vi "RMS.vi"(11 "current waveform":waveform(dbl)) -> (3 "RMS":dbl)   [LabVIEW 2017]
uses:
  <vilib>/measure/madcrms.llb/Basic Averaged DC-RMS for 1 Chan.vi
  <vilib>/measure/NI_MAPro.lvlib
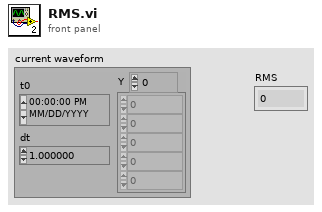
[diagram p1: front panel]
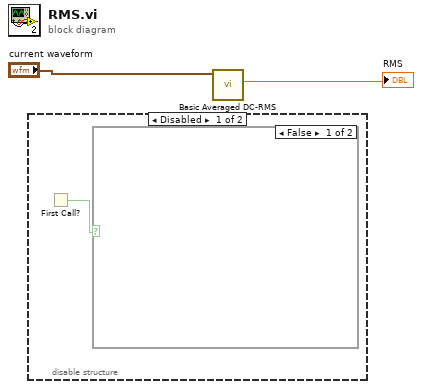
[diagram p0: block diagram]
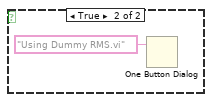
[diagram p2: hidden frame]
diagram:
  n1 = disable-structure shown="Disabled" {
    frame Disabled {
      n2 = First Call?() -> (First Call?: T/F=w3:bool)
      n3 = case shown="False" w3 {
        frame False {
        }
        frame True {
          n4 = One Button Dialog(message="Using Dummy RMS.vi") -> ()  [unwired: 1 in, 1 out]
        }
      }
    }
    frame Enabled {
    }
  }
  n5 = call-poly <vilib>:"Basic Averaged DC-RMS.vi"("signal in"="current waveform") -> ("RMS value"=→"RMS":dbl)  [unwired: 7 in, 3 out]
